vi "Absolute Encoder Open.vi"(11 "Channel":T1) -> (0 "error out":errorcluster, 3 "Cluster":T2)   [LabVIEW 2020]
uses:
  Cluster_Absolute Encoder Ref.ctl
  <vilib>/Rock Robotics/SystemInterfaces/DutyCycle/FPGA_DutyCycleDevRef.ctl
  <vilib>/Rock Robotics/SystemInterfaces/DutyCycle/FPGA_DutyCycleIndex.ctl
  <vilib>/Rock Robotics/WPI/Counter/WPI_CounterDevRef.ctl
  <vilib>/Rock Robotics/SystemInterfaces/Counter/FPGA_CounterCtrSystemIndex.ctl
  <vilib>/Rock Robotics/SystemInterfaces/DIO/FPGA_DIOChannel.ctl
  <vilib>/Rock Robotics/SystemInterfaces/AnalogTrigger/FPGA_AnalogTriggerOutType.ctl
  <vilib>/Rock Robotics/WPI/Counter/WPI_CounterDigitalInputToDigitalSource.vi
  <vilib>/Rock Robotics/WPI/AnalogTrigger/WPI_AnalogTriggerOpen_DutyCycle.vi
  <vilib>/Rock Robotics/WPI/Counter/WPI_CounterAnalogTriggerToDigitalSource.vi
  <vilib>/Rock Robotics/WPI/Counter/WPI_CounterOpen UpDown Mode.vi
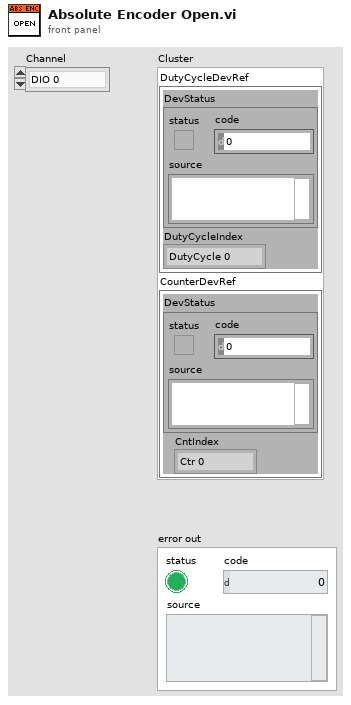
[diagram p1: front panel]
types:
  T1 = typedef "FPGA_DIOChannel.ctl" = enum8{"DIO 0", "DIO 1", "DIO 2", "DIO 3", "DIO 4", "DIO 5", "DIO 6", "DIO 7", "DIO 8", "DIO 9", "DIO MXP 0", "DIO MXP 1", "DIO MXP 2", "DIO MXP 3", "DIO MXP 4", "DIO MXP 5", "DIO MXP 6", "DIO MXP 7", "DIO MXP 8", "DIO MXP 9", "DIO MXP 10", "DIO MXP 11", "DIO MXP 12", "DIO MXP 13", "DIO MXP 14", "DIO MXP 15", "SPI Port CS1", "SPI Port CS2", "SPI Port CS3", "SPI Port MISO", "SPI Port MOSI", "Invalid"}
  T2 = typedef "Cluster_Absolute Encoder Ref.ctl" = cluster{"DutyCycleDevRef":T3, "CounterDevRef":T5}
  T3 = typedef "FPGA_DutyCycleDevRef.ctl" = cluster{"DevStatus":errorcluster, "DutyCycleIndex":T4}
  T4 = typedef "FPGA_DutyCycleIndex.ctl" = enum8{"DutyCycle 0", "DutyCycle 1", "DutyCycle 2", "DutyCycle 3", "DutyCycle 4", "DutyCycle 5", "DutyCycle 6", "DutyCycle 7", "Invalid"}
  T5 = typedef "WPI_CounterDevRef.ctl" = cluster{"DevStatus":errorcluster, "CntIndex":T6}
  T6 = typedef "FPGA_CounterCtrSystemIndex.ctl" = enum8{"Ctr 0", "Ctr 1", "Ctr 2", "Ctr 3", "Ctr 4", "Ctr 5", "Ctr 6", "Ctr 7", "Invalid"}
  T7 = enum16{"Rising Edge", "Falling Edge", "Raising & Falling Edge", "Disabled"}
  T8 = typedef "FPGA_AnalogTriggerOutType.ctl" = enum16{"InWindow", "TriggerState", "Rising", "Falling"}
  T9 = typedef "WPI_DigitalInputDevRef.ctl" = cluster{"DevStatus":errorcluster, "DIO Channel":T1}
  T10 = typedef "FPGA_CounterEncoderSourceConvertionLVSourceType.ctl" = cluster{"DevStatus":errorcluster, "AnalogTriggerMode?":bool, "DigitalMode":cluster{"DIO Channel":T11}, "AnalogTriggerMode":cluster{"AnalogTriggerIndex":T12, "OutputType":T8}}
  T11 = typedef "FPGA_DIODigitalSourceChannel.ctl" = enum8{"DIO 0", "DIO 1", "DIO 2", "DIO 3", "DIO 4", "DIO 5", "DIO 6", "DIO 7", "DIO 8", "DIO 9", "DIO MXP 0", "DIO MXP 1", "DIO MXP 2", "DIO MXP 3", "DIO MXP 4", "DIO MXP 5", "DIO MXP 6", "DIO MXP 7", "DIO MXP 8", "DIO MXP 9", "DIO MXP 10", "DIO MXP 11", "DIO MXP 12", "DIO MXP 13", "DIO MXP 14", "DIO MXP 15", "SPI Port CS1", "SPI Port CS2", "SPI Port CS3", "SPI Port MISO", "SPI Port MOSI", "Disabled"}
  T12 = typedef "FPGA_AnalogTriggerIndex.ctl" = enum8{"Trig 0", "Trig 1", "Trig 2", "Trig 3", "Trig 4", "Trig 5", "Trig 6", "Trig 7", "Invalid"}
  T13 = typedef "FPGA_AnalogTriggerDevRef.ctl" = cluster{"DevStatus":errorcluster, "AnalogTriggerIndex":T12}
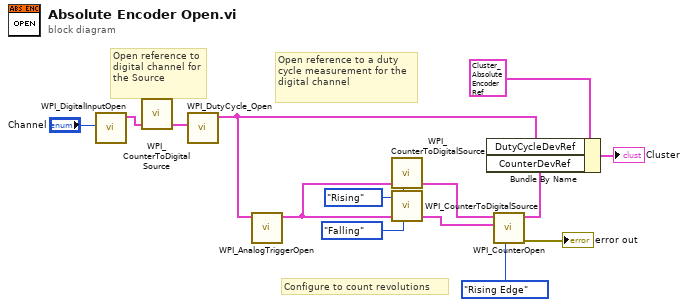
[diagram p0: block diagram]
diagram:
  # "Configure to count revolutions"
  # "Open reference to a duty cycle measurement for the digital channel"
  # "Open reference to digital channel for the Source"
  n1 = call <vilib>:"WPI_DigitalInputOpen.vi"("DIO Channel"="Channel") -> ("DigitalInputDevRef"=w3:T9)  [unwired: 1 in, 9 out]
  n2 = call-poly <vilib>:"WPI_CounterToDigitalSource.vi"("DigitalInputDevRef"=w3) -> ("Digital Source"=w2:T10)  [unwired: 6 out]
  n3 = call <vilib>:"WPI_DutyCycle_Open.vi"("Source"=w2) -> ("DutyCycleDevRef"=w12:T3)  [unwired: 9 in, 1 out]
  n4 = call-poly <vilib>:"WPI_AnalogTriggerOpen.vi"("AnalogTriggerSource"=w12) -> ("AnalogTriggerDevRef"=w9:T13)  [unwired: 9 in, 1 out]
  n5 = call-poly <vilib>:"WPI_CounterToDigitalSource.vi"("AnalogTriggerDevRef"=w9, "OutputType"=FPGA_AnalogTriggerOutType."Rising") -> ("Digital Source"=w5:T10)  [unwired: 5 out]
  n6 = call-poly <vilib>:"WPI_CounterToDigitalSource.vi"("AnalogTriggerDevRef"=w9, "OutputType"=FPGA_AnalogTriggerOutType."Falling") -> ("Digital Source"=w8:T10)  [unwired: 5 out]
  n7 = call-poly <vilib>:"WPI_CounterOpen.vi"("DownEdge"=T7."Rising Edge", "Down Source"=w8, "Up Source"=w5) -> ("error out"=→"error out":errorcluster, "CounterDevRef"=w11:T5)  [unwired: 4 in, 3 out]
  n8 = Bundle By Name(cluster=T2 {"DutyCycleDevRef"={"DevStatus"={"status"=FALSE, "code"=0, "source"=""}, "DutyCycleIndex"=enum."DutyCycle 0"}, "CounterDevRef"={"DevStatus"={"status"=FALSE, "code"=0, "source"=""}, "CntIndex"=enum."Ctr 0"}} ("Cluster"), "DutyCycleDevRef"=w12, "CounterDevRef"=w11) -> (→"Cluster":T2)
